vi "Read database.vi"(0 "table":string="CODMn", 1 "显示项":string[](array[string]), 5 "量程下拉列表":enum16{"低量程", "高量程"}(ring), 7 "历史数据导入":T1(ring), 9 "显示所有数据":bool caption="显示所有数据：", 11 "error in (no error)":errorcluster caption="错误输入（无错误）") -> (4 "表格":string[][](table), 8 "foretime":string, 10 "lasttime":string, 15 "error out":errorcluster caption="错误输出")   [LabVIEW 2016, in "斯坦道CODMn新电路板.lvlib"]
uses:
  <vilib>/addons/database/Connection.llb/DB Tools Open Connec (String).vi
  <vilib>/addons/database/_DB Variant To Data/Database Variant To Data.xnode
  <vilib>/addons/database/NI_Database_API.lvlib
  database/SQLite/SQLite Lib.lvlib
  database/Access/Access Lib.lvlib
panel:
  out "电子表格字符串":string
  out "SQL":string="where 时间 between #2020/03/27 14:26:18 # and #2020/04/26 14:26:18# order by 时间 desc"
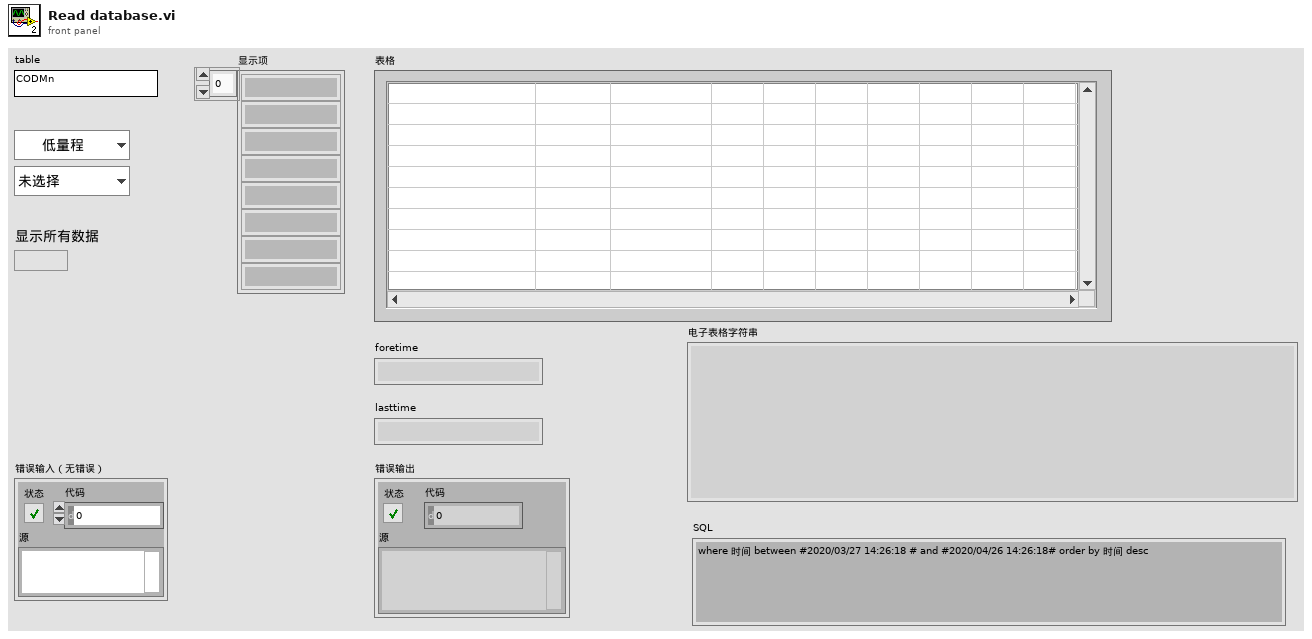
[diagram p1: front panel]
types:
  T1 = enum16{"未选择", "空白校准", "标样校准", "标样核查", "零点核查", "跨度核查"}
  T2 = typedef "数据库类型.ctl" = enum16{"Access", "SQLite"}
  T3 = typedef "NI_Database_API.lvlib/Conn ObjectReference.ctl" = refnum<k1>
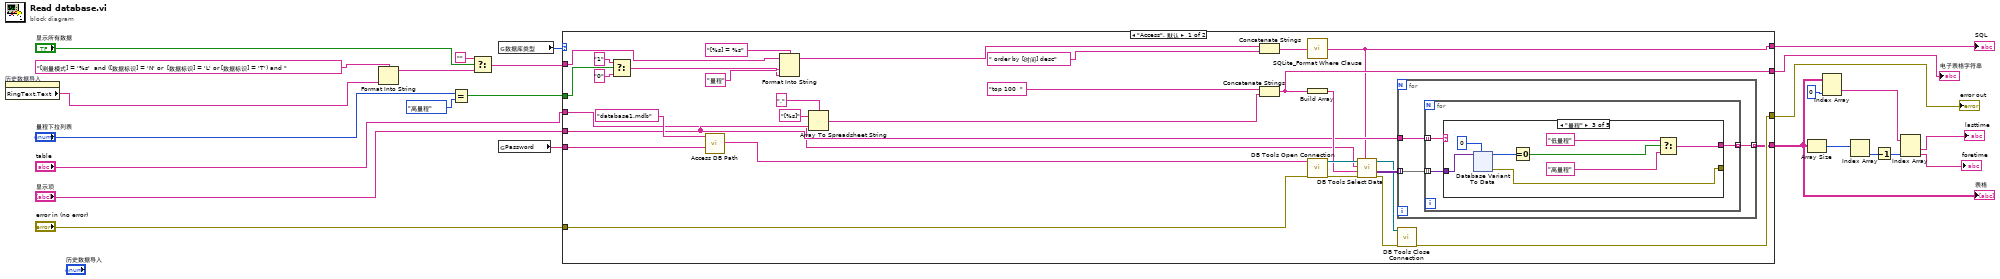
[diagram p0: block diagram]
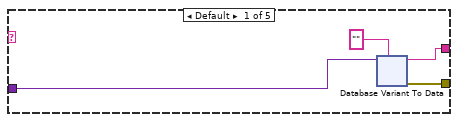
[diagram p2: hidden frame]
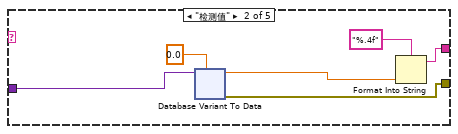
[diagram p3: hidden frame]
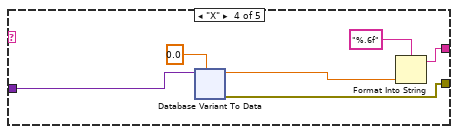
[diagram p4: hidden frame]
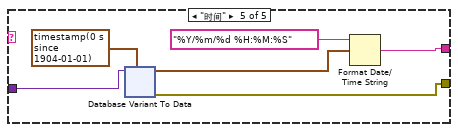
[diagram p5: hidden frame]
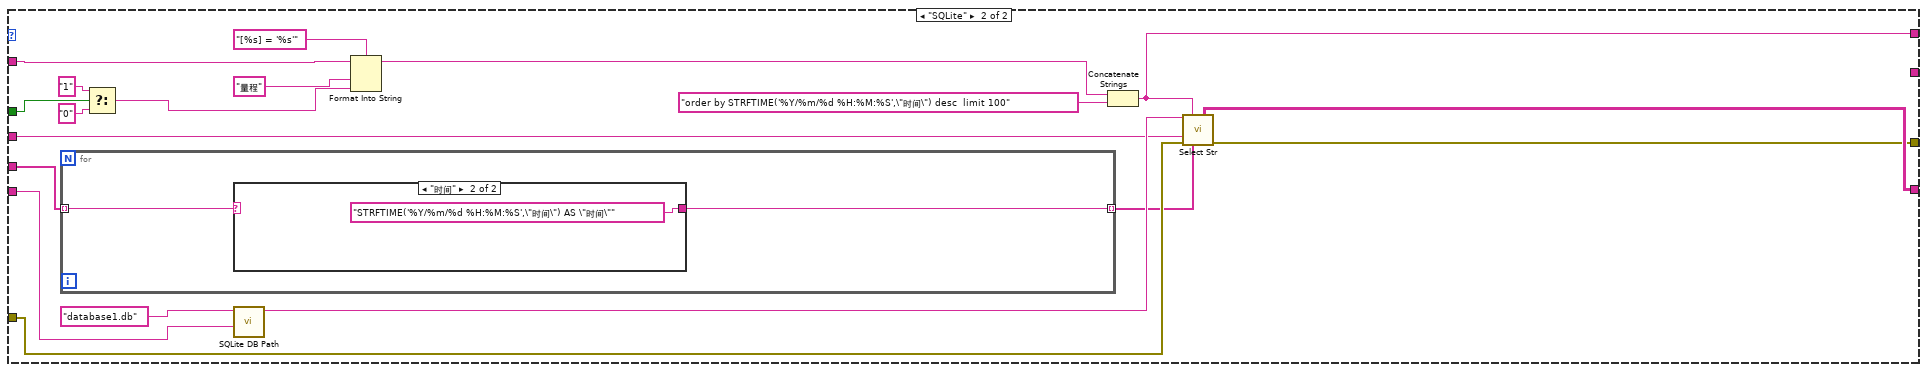
[diagram p6: hidden frame]
diagram:
  n1 = property on="历史数据导入" class="Enum (严格)"() -> ("RingText.Text"=w1:string)  [unwired: 2 in, 2 out]
  n2 = Format Into String(format string="[测量模式] = '%s'  and ([数据标识] = 'N' or  [数据标识] = 'L' or [数据标识] = 'T') and " ("格式字符串"), w1) -> (resulting string=w4:string)  [unwired: 2 in, 1 out]
  n3 = Equal?(x="量程下拉列表", y=enum16{"低量程", "高量程"}."高量程") -> (x = y?=w10:bool)
  n4 = Select(t="", s="显示所有数据", f=w4) -> (s? t:f=w3:string)
  n5 = global read "外部调用接口全局变量.vi" "数据库类型"() -> (w9:T2)
  n6 = global read "外部调用接口全局变量.vi" "Password"() -> (w8:string)
  n7 = case shown="\"Access\", 默认" w9 {
    tunnel: "error in (no error)" -> [w52 w280]
    tunnel: [w51 w279] -> w24
    tunnel: "table" -> [w32 w275]
    tunnel: [w48 w281] -> w17
    tunnel: w3 -> [w36 w271]
    tunnel: "显示项" -> [w40 w278]
    tunnel: [w41 _] -> w18
    tunnel: w10 -> [w30 w274]
    tunnel: w8 -> [w27 w266]
    tunnel: [w26 w265] -> w2
    frame "Access", Default {
      n8 = Select(t="1", s=w30, f="0") -> (s? t:f=w29:string)
      n9 = call "Access DB Path.vi"("Password"=w27, "database"="database1.mdb") -> ("Connection information"=w28:string)  [unwired: 8 in, 1 out]
      n10 = Format Into String(format string="[%s] = %s" ("格式字符串"), initial string=w36, "量程", w29) -> (resulting string=w37:string)  [unwired: 1 in, 1 out]
      n11 = Array To Spreadsheet String(delimiter (Tab)="," ("分隔符(Tab)"), array=w40, 3:"[%s]" ("格式字符串")) -> (spreadsheet string=w45:string)
      n12 = Concatenate Strings(w37, " order by [时间] desc" ("字符串")) -> (w39:string)
      n13 = Concatenate Strings("top 100  " ("字符串"), w45) -> (w41:string)
      n14 = call <userlib>:"SQLite_Format Where Clause.vi"("Where clause"=w39) -> ("String"=w26:string)  [unwired: 4 in]
      n15 = Build Array(w41) -> (w42:string[])
      n16 = call-poly <vilib>:"DB Tools Open Connection.vi"("error in (no error)"=w52, "connection information"=w28) -> ("error out"=w54:errorcluster, "connection reference"=w55:T3)  [unwired: 6 in]
      n17 = call <vilib>:"DB Tools Select Data.vi"("condition"=w26, "error in (no error)"=w54, "columns"=w42, "table"=w32, "connection reference"=w55) -> ("error out"=w53:errorcluster, "data"=w50:variant[][], "connection reference out"=w49:T3)  [unwired: 1 in]
      n18 = for {
        tunnel: w50 -> [w58] mode=indexing
        tunnel: [w57] -> w48 mode=indexing
        tunnel: w40 -> [w56]
        n19 = for {
          tunnel: w58 -> [w60] mode=indexing
          tunnel: [w61] -> w57 mode=indexing
          tunnel: w56 -> [w59] mode=indexing
          n20 = case shown="\"量程\"" w59 {
            tunnel: w60 -> [w65 w103 w143 w181 w219]
            tunnel: [w62 w99 w138 w177 w215] -> w61
            tunnel: [w63 w102 w142 w180 w214] -> _
            frame Default {
              n21 = xnode "Database Variant To Data"("database variant"=w65, "type"="") -> ("data"=w62:string, "error out"=w63:errorcluster)  [unwired: 1 in]
            }
            frame "检测值" {
              n22 = xnode "Database Variant To Data"("database variant"=w103, "type"=0.0) -> ("data"=w100:dbl, "error out"=w102:errorcluster)  [unwired: 1 in]
              n23 = Format Into String(format string="%.4f" ("格式字符串"), w100) -> (resulting string=w99:string)  [unwired: 2 in, 1 out]
            }
            frame "量程" {
              n24 = xnode "Database Variant To Data"("database variant"=w143, "type"=u8 0) -> ("data"=w140:u8, "error out"=w142:errorcluster)  [unwired: 1 in]
              n25 = Equal To 0?(x=w140) -> (x = 0?=w139:bool)
              n26 = Select(t="低量程", s=w139, f="高量程") -> (s? t:f=w138:string)
            }
            frame "X" {
              n27 = xnode "Database Variant To Data"("database variant"=w181, "type"=0.0) -> ("data"=w178:dbl, "error out"=w180:errorcluster)  [unwired: 1 in]
              n28 = Format Into String(format string="%.6f" ("格式字符串"), w178) -> (resulting string=w177:string)  [unwired: 2 in, 1 out]
            }
            frame "时间" {
              n29 = xnode "Database Variant To Data"("database variant"=w219, "type"=timestamp(0 s since 1904-01-01) ("当前时间")) -> ("data"=w218:timestamp, "error out"=w214:errorcluster)  [unwired: 1 in]
              n30 = Format Date/Time String(time format string (%c)="%Y/%m/%d %H:%M:%S" ("时间格式字符串(%c)"), seconds (now)=w218) -> (date/time string=w215:string)  [unwired: 1 in]
            }
          }
        }
      }
      n31 = call <vilib>:"DB Tools Close Connection.vi"("error in (no error)"=w53, "connection reference"=w49) -> ("error out"=w51:errorcluster)  [unwired: 5 in]
    }
    frame "SQLite" {
      n32 = for {
        tunnel: w278 -> [w285] mode=indexing
        tunnel: [w284] -> w277 mode=indexing
        n33 = case shown="\"时间\"" w285 {
          selector: w285 -> [w286 _]
          tunnel: [w286 "STRFTIME('%Y/%m/%d %H:%M:%S',\"时间\") AS \"时间\""] -> w284
          frame Default {
          }
          frame "时间" {
          }
        }
      }
      n34 = Select(t="1", s=w274, f="0") -> (s? t:f=w269:string)
      n35 = call "SQLite DB Path.vi"("Password"=w266, "database"="database1.db") -> ("Path out"=w282:string)  [unwired: 9 in]
      n36 = Format Into String(format string="[%s] = '%s'" ("格式字符串"), initial string=w271, "量程", w269) -> (resulting string=w267:string)  [unwired: 1 in, 1 out]
      n37 = Concatenate Strings(w267, "order by STRFTIME('%Y/%m/%d %H:%M:%S',\"时间\") desc  limit 100") -> (w265:string)
      n38 = call "Select Str.vi"("DB Path"=w282, "Where Clause"=w265, "Tables Name"=w275, "error in (no error)"=w280, "Columns"=w277) -> ("Results"=w281:string[][], "error out"=w279:errorcluster)  [unwired: 7 in, 2 out]
    }
  }
  "表格" <- w17
  "error out" <- w24
  "SQL" <- w2
  "电子表格字符串" <- w18
  n39 = Array Size(array=w17) -> (size(s)=w16:i32[])
  n40 = Index Array(array=w17, index (col)=0 ("禁用的索引 (列)")) -> (element=w22:string[])  [unwired: 1 in]
  n41 = Index Array(array=w16) -> (element=w15:i32)  [unwired: 1 in]
  n42 = Decrement(x=w15) -> (x-1=w14:i32)
  n43 = Index Array(array=w22, index #2=w14) -> (element #1=→"lasttime":string, element #2=→"foretime":string)  [unwired: 1 in]
